vi "Alarm Monitor.vi"(8 "error in (no error)":errorcluster, 10 "Alarm":refnum<notifier>, 11 "Sound file":path) -> (0 "error out":errorcluster)   [LabVIEW 2024]
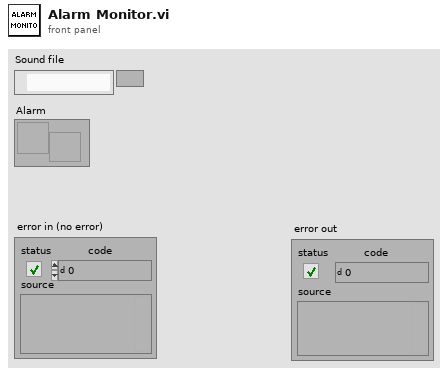
[diagram p1: front panel]
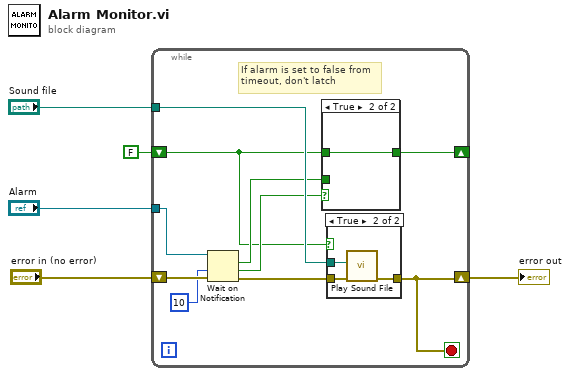
[diagram p0: block diagram]
diagram:
  n1 = while {
    tunnel: "Alarm" -> [w14]
    shift-right: [w12] -> w4
    shift-left: "error in (no error)" -> [w15]
    tunnel: "Sound file" -> [w11]
    shift-right: [w6] -> _
    shift-left: FALSE -> [w7]
    stop <- w12 stop-if-true
    # "If alarm is set to false from\ntimeout, don't latch"
    n2 = Wait on Notification(notifier=w14, timeout in ms (-1)=10, error in (no error)=w15) -> (notification=w9:bool, timed out?=w8:bool, error out=w13:errorcluster)  [unwired: 1 in, 1 out]
    n3 = case shown="True" w8 {
      tunnel: w9 -> [w16 _]
      tunnel: w7 -> [_ w17]
      tunnel: [w16 w17] -> w6
      frame False {
      }
      frame True {
      }
    }
    n4 = case shown="True" w7 {
      tunnel: w13 -> [w18 w21]
      tunnel: [w18 w20] -> w12
      tunnel: w11 -> [_ w19]
      frame False {
      }
      frame True {
        n5 = call <vilib>:"Play Sound File.vi"("error in (no error)"=w21, "path"=w19) -> ("error out"=w20:errorcluster)  [unwired: 8 in, 1 out]
      }
    }
  }
  "error out" <- w4
